vi "GoPro Make Authed Request.vi"(8 "error in (no error)":errorcluster, 9 "Params":T3[](array[typedef]), 10 "url":string, 11 "Gopro DevRef":T1) -> (0 "error out":errorcluster, 1 "body":string, 2 "headers":string, 3 "Output DevRef":T1)   [LabVIEW 2015]
uses:
  GET Parameter.ctl
  GoPro DevRef.ctl
  <vilib>/httpClient/ClientHandle.ctl
  <vilib>/httpClient/LabVIEWHTTPClient.lvlib
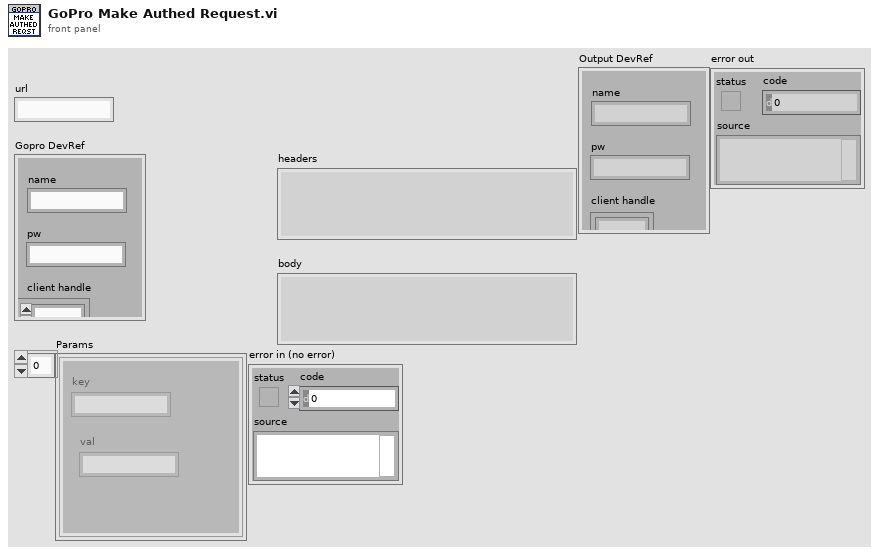
[diagram p1: front panel]
types:
  T1 = typedef "GoPro DevRef.ctl" = cluster{"name":string, "pw":string, "client handle":T2}
  T2 = typedef "LabVIEWHTTPClient.lvlib/ClientHandle.ctl" = refnum<k1>
  T3 = typedef "GET Parameter.ctl" = cluster{"key":string, "val":string}
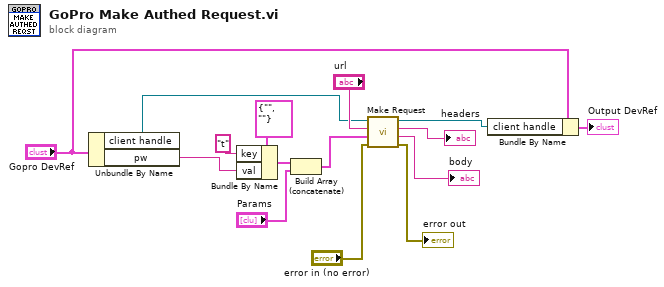
[diagram p0: block diagram]
diagram:
  n1 = Unbundle By Name("Gopro DevRef") -> ("client handle"=w12:T2, "pw"=w8:string)
  n2 = Bundle By Name(cluster=T3 {"key"="", "val"=""} ("GET Parameter"), "key"="t", "val"=w8) -> (w9:T3)
  n3 = Build Array (concatenate)(w9, "Params") -> (w10:T3[])
  n4 = call "Make Request.vi"("error in (no error)"="error in (no error)", "Parameters"=w10, "url"="url", "Refnum in"=w12) -> ("error out"=→"error out":errorcluster, "body"=→"body":string, "headers"=→"headers":string, "client handle out"=w4:T2)  [unwired: 4 in]
  n5 = Bundle By Name(cluster="Gopro DevRef", "client handle"=w4) -> (→"Output DevRef":T1)
